vi "CloseFile.vi"(8 "error in (no error)":errorcluster, 11 "ExistingFileMgr in":refnum<class "ExistingFileMgr.lvclass">) -> (0 "error out":errorcluster, 3 "ExistingFileMgr out":refnum<class "ExistingFileMgr.lvclass">)   [LabVIEW 2019, in "ExistingFileMgr.lvclass"]
uses:
  ExistingFileMgr.lvclass
  ExistingFileMgr.lvclass/ExistingFileMgr.ctl
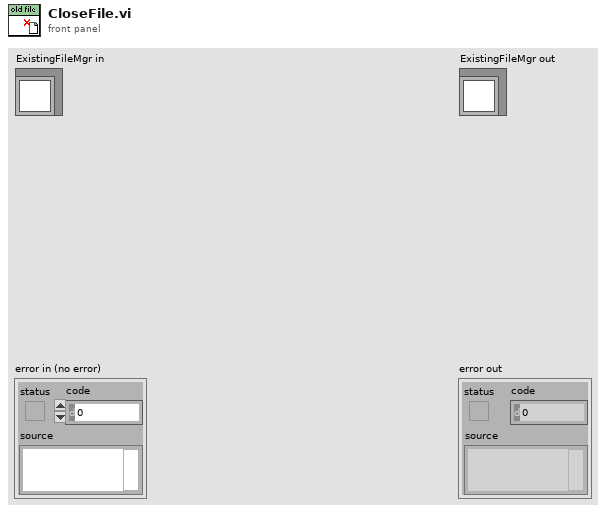
[diagram p1: front panel]
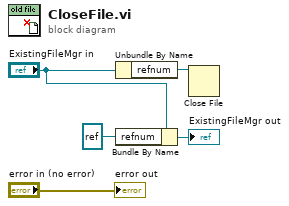
[diagram p0: block diagram]
diagram:
  n1 = Unbundle By Name("ExistingFileMgr in") -> ("refnum"=w5:refnum<file>)
  n2 = Bundle By Name(cluster="ExistingFileMgr in", "refnum"=refnum<file> refnum) -> (→"ExistingFileMgr out":refnum<class "ExistingFileMgr.lvclass">)
  n3 = Close File(refnum=w5) -> ()  [unwired: 1 in, 2 out]
  "error out" <- "error in (no error)"
